vi "remove_redundant_open_brace.vi"(8 "error in (no error)":errorcluster, 11 "Instrument Command In":string) -> (0 "error out":errorcluster, 3 "Instrument Command Out":string)   [LabVIEW 2018]
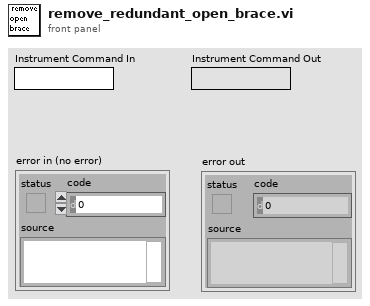
[diagram p1: front panel]
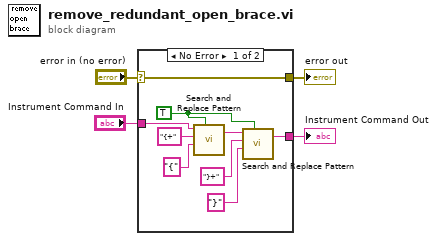
[diagram p0: block diagram]
diagram:
  n1 = case shown="No Error" "error in (no error)" {
    selector: "error in (no error)" -> [w5 w15]
    tunnel: [w12 w14] -> w4
    tunnel: "Instrument Command In" -> [w11 w14]
    tunnel: [w5 w15] -> w1
    frame No Error {
      w13 = TRUE
      n2 = call <vilib>:"Search and Replace Pattern.vi"("string"=w11, "regular expression (\"\")"="{+" ("regular expression (\"\")"), "replace string (\"\")"="{" ("replace string (\"\")"), "replace all? (F)"=w13) -> ("result string"=w8:string)  [unwired: 2 out]
      n3 = call <vilib>:"Search and Replace Pattern.vi"("string"=w8, "regular expression (\"\")"="}+" ("regular expression (\"\")"), "replace string (\"\")"="}" ("replace string (\"\")"), "replace all? (F)"=w13) -> ("result string"=w12:string)  [unwired: 2 out]
    }
    frame Error {
    }
  }
  "Instrument Command Out" <- w4
  "error out" <- w1
